vi "Convert Fcurve units.vi"(0 "reference in":refnum<class "XYgraph.lvclass">, 5 "error in (no error)":errorcluster, 9 "X scale Offset":dbl, 11 "Y scale Offset":dbl) -> (14 "reference out":refnum<class "XYgraph.lvclass">, 19 "error out":errorcluster)   [LabVIEW 2019, in "XYgraph.lvclass"]
doc: "Converts the Force curve units using the provided metadata"
uses:
  XYgraph.lvclass
  <vilib>/Utility/miscctls.llb/LVOffsetAndMultiplierTypeDef.ctl
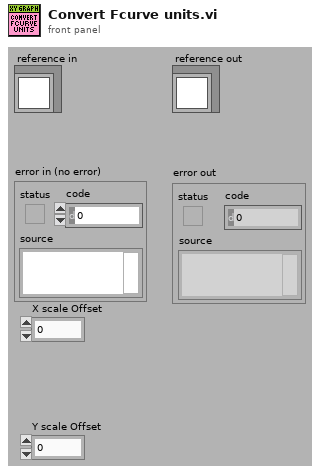
[diagram p1: front panel]
types:
  T1 = typedef "LVOffsetAndMultiplierTypeDef.ctl" = cluster{"Offset":dbl, "Multiplier":dbl}
  T2 = typedef "XYgraph.lvclass/ObjectAttributesRef.ctl" = refnum<data-value>
  T3 = typedef "XYgraph.lvclass/ObjectAttributes.ctl" = cluster{"FPref":T4, "MyAttribute":dbl, "X multiplier":dbl, "Y multiplier":dbl, "X Scale name":string, "Y Scale name":string, "Fcurve metadata":T5, "Fcurve":refnum<class "Fcurve.lvclass">}
  T4 = typedef "XYgraph.lvclass/XY graph ref.ctl" = refnum<vi>
  T5 = typedef "Fcurve.lvclass/Metadata.ctl" = cluster{"dt (us)":dbl, "Dec Factor":dbl, "Z piezo Sensitivity (nm/V)":dbl, "K (N/m)":dbl, "Sp (V)":dbl, "Contact (ms)":dbl, "Zpos contact":dbl, "Vel_app (nm/s)":dbl, "Vel_ret (nm/s)":dbl, "deltaV (nm)":dbl, "Def_V0 (v)":dbl, "Piezo gain":dbl, "invOLS (nm/V)":dbl}
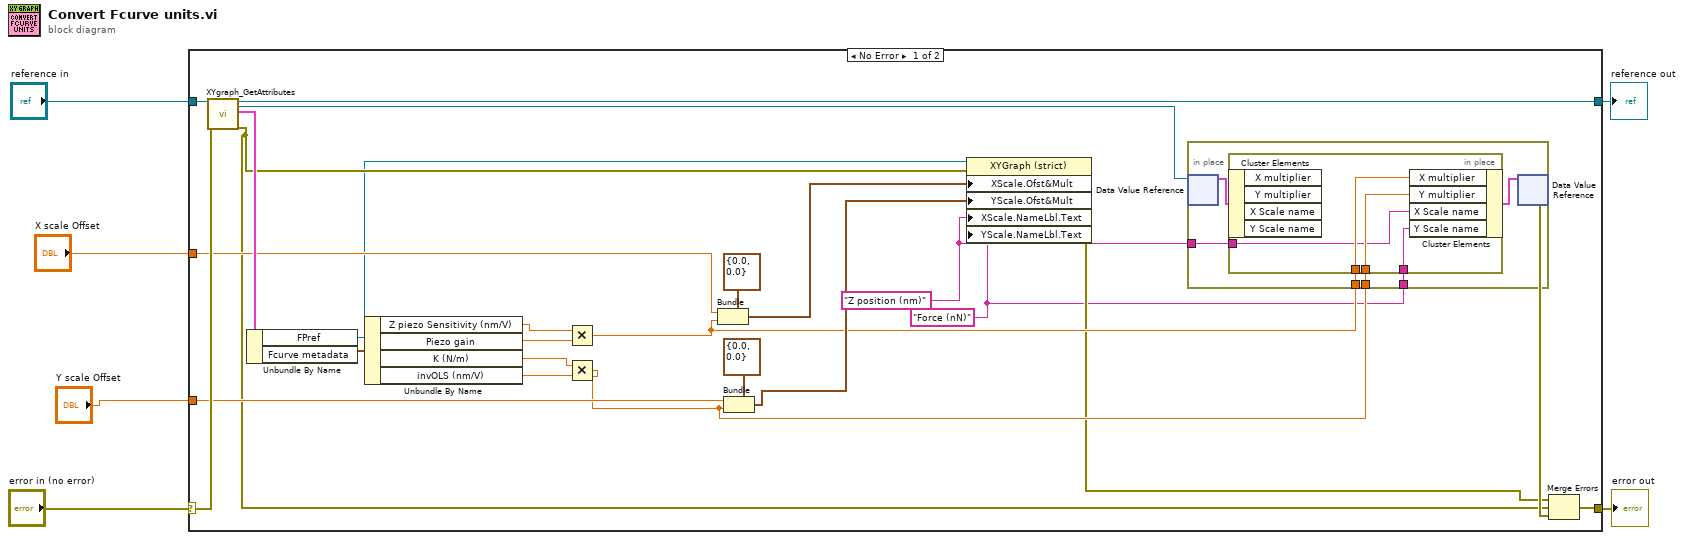
[diagram p0: block diagram]
diagram:
  n1 = case shown="No Error" "error in (no error)" {
    selector: "error in (no error)" -> [w31 w43]
    tunnel: [w17 w43] -> w5
    tunnel: [w9 w42] -> w3
    tunnel: "reference in" -> [w29 w42]
    tunnel: "Y scale Offset" -> [w23 _]
    tunnel: "X scale Offset" -> [w22 _]
    frame No Error {
      w11 = "Force (nN)" ("Y Scale.Name Label.Text")
      w12 = "Z position (nm)" ("X Scale.Name Label.Text")
      n2 = call "XYgraph_GetAttributes.vi"("reference in"=w29, "error in (no error)"=w31) -> ("reference out"=w9:refnum<class "XYgraph.lvclass">, "attributes ref"=w16:T2, "attributes"=w30:T3, "error out"=w8:errorcluster)  [unwired: 14 in]
      n3 = Unbundle By Name(w30) -> ("FPref"=w7:T4, "Fcurve metadata"=w10:T5)
      n4 = Unbundle By Name(w10) -> ("Z piezo Sensitivity (nm/V)"=w28:dbl, "Piezo gain"=w27:dbl, "K (N/m)"=w21:dbl, "invOLS (nm/V)"=w20:dbl)
      n5 = Multiply(x=w28, y=w27) -> (x*y=w15:dbl)
      n6 = Multiply(x=w21, y=w20) -> (x*y=w14:dbl)
      n7 = Bundle(cluster=T1 {"Offset"=0.0, "Multiplier"=0.0} ("X Scale.Offset and Multiplier"), "Offset"=w22, "Multiplier"=w15) -> (w26:T1)
      n8 = Bundle(cluster=T1 {"Offset"=0.0, "Multiplier"=0.0} ("Y Scale.Offset and Multiplier"), "Offset"=w23, "Multiplier"=w14) -> (w19:T1)
      n9 = property on="Property Node" class="XYGraph (strict)"(reference=w7, error in=w8, "XScale.Ofst&Mult"=w26, "YScale.Ofst&Mult"=w19, "XScale.NameLbl.Text"=w12, "YScale.NameLbl.Text"=w11) -> (error out=w13:errorcluster)  [unwired: 1 out]
      n10 = in-place {
        in-place-border: w15 -> [w35]
        in-place-border: w14 -> [w34]
        in-place-border: w12 -> [w33]
        in-place-border: w11 -> [w32]
        n11 = in-place-dvr #1(w16) -> (w36:T3)  [unwired: 1 out]
        n12 = in-place {
          in-place-border: w35 -> [w41]
          in-place-border: w34 -> [w40]
          in-place-border: w33 -> [w39]
          in-place-border: w32 -> [w38]
          n13 = in-place-cluster #2(w36) -> ()  [unwired: 4 out]
          n14 = in-place-cluster #2("X multiplier"=w41, "Y multiplier"=w40, "X Scale name"=w39, "Y Scale name"=w38) -> (w37:T3)
        }
        n15 = in-place-dvr #1(w37) -> (w18:errorcluster)  [unwired: 1 out]
      }
      n16 = Merge Errors(w13, w8, w18) -> (w17:errorcluster)
    }
    frame Error {
    }
  }
  "error out" <- w5
  "reference out" <- w3
